vi "Apply move.vi"(8 "error in (no error)":errorcluster, 10 "Position in":refnum<class "Position.lvclass">, 11 "Move in":refnum<class "Move.lvclass">) -> (0 "error out":errorcluster, 2 "Position out":refnum<class "Position.lvclass">, 3 "Move out":refnum<class "Move.lvclass">)   [LabVIEW 2015, in "Chesslib.lvlib" / "Move.lvclass"]
uses:
  Move.lvclass
  Position/Position.lvclass
  typedef/Piece type.ctl
  Move.lvclass/Move.ctl
  Position/Position.lvclass/Position.ctl
  Pieces/Piece/Piece.lvclass
  Board/Board.lvclass
  Chesslib.lvlib
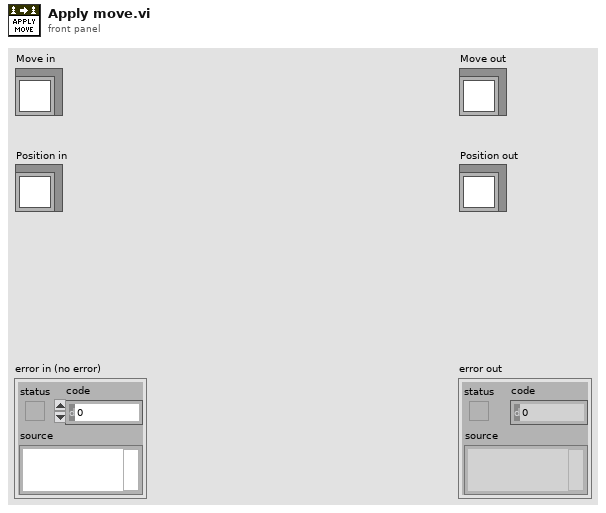
[diagram p1: front panel]
types:
  T1 = typedef "Chesslib.lvlib/Piece type.ctl" = enum16{"Pawn", "Bishop", "Knight", "Rook", "Queen", "King"}
  T2 = typedef "Chesslib.lvlib/Square.ctl" = cluster{"File":T3, "Rank":T4}
  T3 = typedef "Chesslib.lvlib/File.ctl" = enum8{"a", "b", "c", "d", "e", "f", "g", "h"}
  T4 = typedef "Chesslib.lvlib/Rank.ctl" = enum8{"1", "2", "3", "4", "5", "6", "7", "8"}
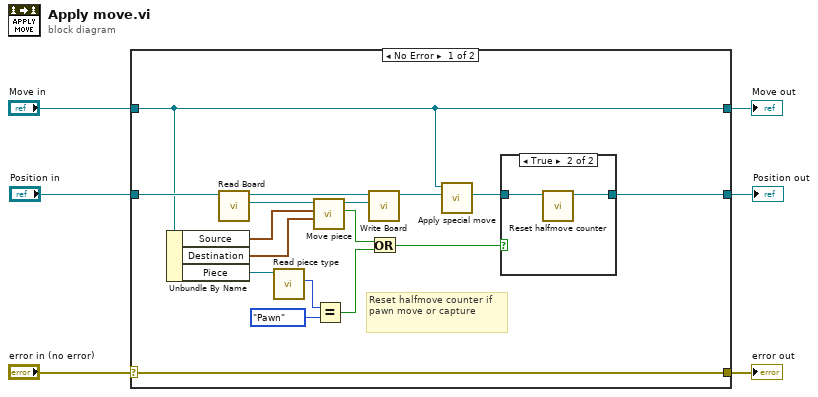
[diagram p0: block diagram]
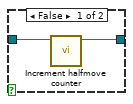
[diagram p2: hidden frame]
diagram:
  n1 = case shown="No Error" "error in (no error)" {
    selector: "error in (no error)" -> [w23 w30]
    tunnel: [w23 w30] -> w5
    tunnel: [w14 w29] -> w3
    tunnel: "Move in" -> [w14 w29]
    tunnel: [w8 w28] -> w2
    tunnel: "Position in" -> [w22 w28]
    frame No Error {
      # "Reset halfmove counter if pawn move or capture"
      n2 = Unbundle By Name(w14) -> ("Source"=w17:T2, "Destination"=w16:T2, "Piece"=w13:refnum<class "Piece.lvclass">)
      n3 = call "Read Board.vi"("Position in"=w22) -> ("Chesslib.lvlib:Board.lvclass"=w19:refnum<class "Board.lvclass">, "Position out"=w21:refnum<class "Position.lvclass">)  [unwired: 9 in]
      n4 = call-dynamic "Read piece type.vi"("Piece in"=w13) -> ("Piece type"=w11:T1)  [unwired: 10 in]
      n5 = call "Move piece.vi"("Destination"=w16, "Source"=w17, "Board in"=w19) -> ("Destination occupied?"=w12:bool, "Board out"=w18:refnum<class "Board.lvclass">)  [unwired: 6 in, 1 out]
      n6 = Equal?(x=w11, y=Piece_type."Pawn") -> (x = y?=w9:bool)
      n7 = call "Write Board.vi"("Board"=w18, "Position in"=w21) -> ("Position out"=w20:refnum<class "Position.lvclass">)  [unwired: 9 in]
      n8 = Or(x=w12, y=w9) -> (x .or. y?=w7:bool)
      n9 = call-dynamic "Apply special move.vi"("Position in"=w20, "Move in"=w14) -> ("Position out"=w15:refnum<class "Position.lvclass">)  [unwired: 7 in, 2 out]
      n10 = case shown="True" w7 {
        tunnel: w15 -> [w25 w27]
        tunnel: [w24 w26] -> w8
        frame False {
          n11 = call "Increment halfmove counter.vi"("Position in"=w25) -> ("Position out"=w24:refnum<class "Position.lvclass">)  [unwired: 9 in, 1 out]
        }
        frame True {
          n12 = call "Reset halfmove counter.vi"("Position in"=w27) -> ("Position out"=w26:refnum<class "Position.lvclass">)  [unwired: 9 in, 1 out]
        }
      }
    }
    frame Error {
    }
  }
  "error out" <- w5
  "Move out" <- w3
  "Position out" <- w2
